vi "Poly.vi"   [LabVIEW 2022 SP3]
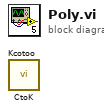
[diagram p0: block diagram]
diagram:
  n1 = call "CtoK.vi"() -> ()  [unwired: 11 in, 1 out]
  n2 = call "Kcotoo.vi"() -> ()  [unwired: 11 in, 1 out]
